vi "5ChPulserTrigsNew.vi"(1 "Motion Settings":T1={"No Motion?"=FALSE, "Motion System"=enum."NI 735x", "Motion Bd ID"=1, "Motion Profile"="SMAC1", "# Axis"=1, "Reverse Z axis?"=TRUE, "SMAC Axis"=0, "scan pair"=enum."y-(x) scan", "RT fps"=6.0, "Steps per mm"=[1000, 1000, 1000, 1000], "Motor Parameters"={"velocity ct/s"=[10000.0, 10000.0, 10000.0, 50000.0], "accel ct/s^2"=[50000.0, 50000.0, 50000.0, 200000.0]}, "One Way Scan"=FALSE, "Reverse One Way Scan"=FALSE, "Global Position (mm)"=[], "Plane"=0, "Distance between\nscan lines (um)"=0.0, "Distance between\nscan planes (um)"=0.0, "number of scan planes"=1, "Total steps in line"=0, "Xtra plane\ndistance  (um)"=100, "Xtra planes "=1, "Add Axis"=FALSE, "overshoot cts"=200, "BKPT Shift"=0, "Scan Start Time (ms)"=0, "ESP VISA"="GPIB::1::INSTR", "3rd Axis"=1, "GL Ref Out"=refnum, "Galil Address"=""} {"3rd Axis" items=["x", "y", "z", "w"]; "Xtra planes" min=1; "Xtra plane\ndistance  (um)" min=0; "Distance between\nscan planes (um)" format="%.2f"; "Distance between\nscan lines (um)" format="%.2f"; "SMAC Axis" items=["None"=0, "Axis 1"=1, "Axis 2"=2, "Axis 3"=3, "Axis 4"=4, "Axis 5"=5, "Axis 6"=6, "Axis 7"=7, "Axis 8"=8, "Vector Space 1"=17, "Vector Space 2"=18, "Vector Space 3"=19, "Vector Space 4"=20]; "Motion Bd ID" min=1 max=32 step=1}, 5 "Digitizer Settings":T5={"Digitizer delay (us) "=0.0, "rf points per line"=2048, "lines per plane"=128, "Samp Rate (Hz)"=100000000.0, "Additional dig delay (us)"=0.0, "Voltage Scale"=0.4, "Pre-Looks"=0, "Offset delay (us)"=0.0, "bits A/D"=8, "Avg Num"=1, "DigTimeOut"=5.0, "Rel Dig Delay"=0.0, "Dig Ch"=0, "LeCroyCluster"={"LeCroy Channels"=[TRUE, FALSE, FALSE, FALSE], "LC read pt offset"=0.0, "Sweep Avg"=FALSE}, "Main Digitizer"=enum."NI Digitizer", "Dig Config"=enum."Single channel", "Digitizer ID Cluster"={"Acqiris/Alazar/SP ID"=[], "NI Instr Handles"=[], "LeCroy VISA"="", "GaGe Handle"={"Handle"=0, "Sample size"=0, "Resolution"=0, "Offset"=0, "Channels"=0, "Boards"=0}, "ATS Ref"="ATS9350", "Acqiris Address"=["PCI::INSTR0"], "ADQRef"=refnum, "adq_cu_ptr"=refnum}, "Trigger Settings"={"Trig Source"=1, "Trig Coupling"=0, "Trig Slope"=0, "Level (mV)"=1500.0}, "Bulk Acq"=FALSE, "Bulk Start Indexes"=[], "Data Ref RF"=refnum, "NI ID/Channel"=[], "Total Dig CH"=1, "Xtra Ann Trig delay (us)"=10.0, "Fix Z Delay?"=FALSE, "One Way Transmission?"=FALSE, "Data Ref Log"=refnum} {"Trigger Settings"."Trig Slope" items=["Positive", "Negative"]; "Trigger Settings"."Level (mV)" format="%.2f"; "Trigger Settings"."Trig Coupling" items=["DC 1 MOhm", "AC 1 MOhm", "DC 50 Ohm", "AC 50 Ohm"]; "Trigger Settings"."Trig Source" items=["Chan 1", "External"]; "Rel Dig Delay" format="%.2f"; "DigTimeOut" format="%.2f"; "Avg Num" min=1; "Offset delay (us)" format="%.2f"; "Additional dig delay (us)" format="%.2f"; "Digitizer delay (us)" format="%.2f"}, 6 "XMIT":bool[](array[boolean])=[TRUE, TRUE, TRUE, TRUE, TRUE], 7 "high time":dbl=1e-06 format="%^.2e", 8 "Axis":u16(ring)=1 caption="Axis or Vector Space" items=["Axis 1"=1, "Axis 2"=2, "Axis 3"=3, "Axis 4"=4, "Axis 5"=5, "Axis 6"=6, "Axis 7"=7, "Axis 8"=8, "Vector Space 1"=17, "Vector Space 2"=18, "Vector Space 3"=19, "Vector Space 4"=20], 9 "M-mode?":bool, 10 "error in":errorcluster) -> (0 "5CH Pulser Tasks":refnum<k21>[](array[refnum]), 3 "error out":errorcluster)   [LabVIEW 2022 SP3]
uses:
  Digitizers/-DigitizerRoutines/DigitizerSettings.ctl
  Digitizers/-DigitizerRoutines/Digitizer.ctl
  Digitizers/-DigitizerRoutines/DigConfig.ctl
  Digitizers/-DigitizerRoutines/DigitizerID.ctl
  C:/Windows/System32/ADQAPI_dotNet_helper.dll
  Windows/System32/ADQAPI_dotNet_helper.dll
  Motion Controllers/NI_controller/-NI_MotionRoutines/MotionParameters.ctl
  Motion Controllers/NI_controller/-NI_MotionRoutines/MotionSys.ctl
  Motion Controllers/-MotionRoutines/ScanAxis.ctl
  Motion Controllers/-MotionRoutines/3rdAxis.ctl
  Switch Modules/SwitchGlobals.vi
  Motion Controllers/-MotionRoutines/MotionGlobals.vi
  <vilib>/DAQmx/create/channels.llb/DAQmx Create Channel (CO-Pulse Generation-Time).vi
  <vilib>/DAQmx/configure/trigger.llb/DAQmx Start Trigger (Digital Edge).vi
  PulserGlobals.vi
  <vilib>/DAQmx/create/channels.llb/DAQmx Create Channel (CO-Pulse Generation-Frequency).vi
  <vilib>/DAQmx/configure/timing.llb/DAQmx Timing (Implicit).vi
  <resource>/objmgr/daqmx.rc
panel:
  out "Array":dbl[](array[numeric]) format="%#_3e"
  in  "stop":bool
  # "Counter 1 output is the BNC on grey box."
  # "Trigger source comes from Gate of CTR0 (PFI9)\n\nThe NI trigger connector routes to CTR0 Gate"
  # "1-D and 2-D B scan settings"
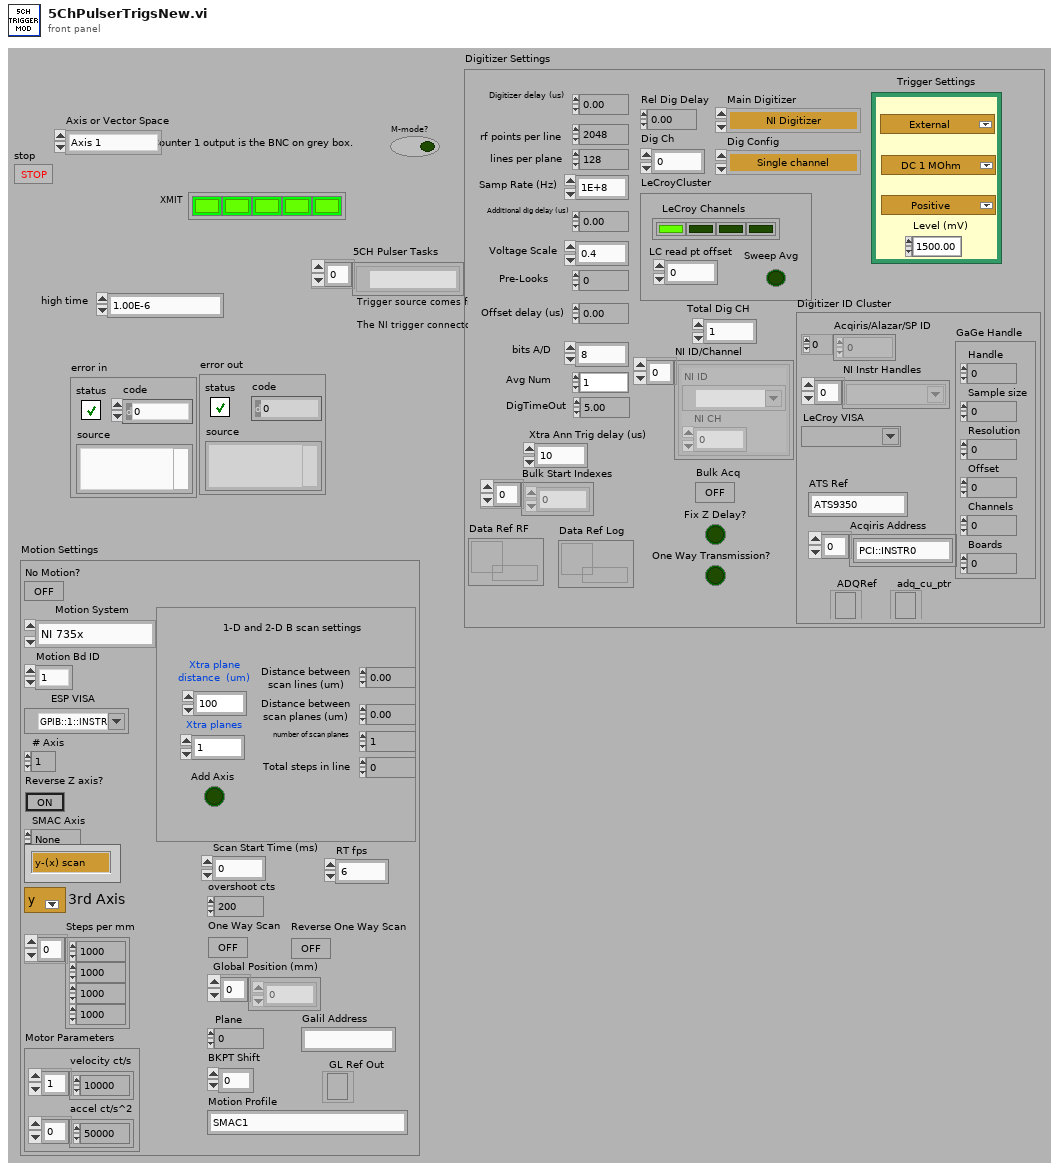
[diagram p1: front panel]
types:
  T1 = typedef "MotionParameters.ctl" = cluster{"No Motion?":bool, "Motion System":T2, "Motion Bd ID":u8, "Motion Profile":string, "# Axis":i8, "Reverse Z axis?":bool, "SMAC Axis":u16, "scan pair":T3, "RT fps":sgl, "Steps per mm":i32[], "Motor Parameters":cluster{"velocity ct/s":dbl[], "accel ct/s^2":dbl[]}, "One Way Scan":bool, "Reverse One Way Scan":bool, "Global Position (mm)":dbl[], "Plane":i32, "Distance between\nscan lines (um)":sgl, "Distance between\nscan planes (um)":sgl, "number of scan planes":i32, "Total steps in line":i32, "Xtra plane\ndistance  (um)":i32, "Xtra planes ":i32, "Add Axis":bool, "overshoot cts":i32, "BKPT Shift":i32, "Scan Start Time (ms)":u32, "ESP VISA":refnum<visa-resource-name>, "3rd Axis":T4, "GL Ref Out":refnum<k7>, "Galil Address":string}
  T2 = typedef "MotionSys.ctl" = enum16{"MM3000", "NI 735x", "Newport ESP", "No Motion Card", "Galil"}
  T3 = typedef "ScanAxis.ctl" = enum16{"y-(x) scan", "x-(y) scan", "z-(x) scan", "z-(y) scan", "y-(z) scan", "x-(z) scan", "w-(x) scan", "w-(y) scan", "w-(z) scan", "x-(w) scan", "y-(w) scan", "z-(w) scan"}
  T4 = typedef "3rdAxis.ctl" = u16
  T5 = typedef "DigitizerSettings.ctl" = cluster{"Digitizer delay (us) ":dbl, "rf points per line":i32, "lines per plane":i32, "Samp Rate (Hz)":dbl, "Additional dig delay (us)":dbl, "Voltage Scale":dbl, "Pre-Looks":i32, "Offset delay (us)":dbl, "bits A/D":i8, "Avg Num":i32, "DigTimeOut":sgl, "Rel Dig Delay":sgl, "Dig Ch":i32, "LeCroyCluster":cluster{"LeCroy Channels":bool[], "LC read pt offset":dbl, "Sweep Avg":bool}, "Main Digitizer":T6, "Dig Config":T7, "Digitizer ID Cluster":T8, "Trigger Settings":cluster{"Trig Source":u16, "Trig Coupling":u16, "Trig Slope":u16, "Level (mV)":dbl}, "Bulk Acq":bool, "Bulk Start Indexes":i32[], "Data Ref RF":refnum<data-value>, "NI ID/Channel":cluster{"NI ID":refnum<k15>, "NI CH":i32}[], "Total Dig CH":i32, "Xtra Ann Trig delay (us)":dbl, "Fix Z Delay?":bool, "One Way Transmission?":bool, "Data Ref Log":refnum<data-value>}
  T6 = typedef "Digitizer.ctl" = enum16{"Acqiris Digitizer", "NI Digitizer", "LeCroy", "GaGe", "AlazarTech", "No Digitizer", "Teledyne"}
  T7 = typedef "DigConfig.ctl" = enum16{"Single channel", "2 Chans w/ 2 Acqiris", "2 Chans w/ 1 Acqiris", "5-CH Pulser New", "5-CH pulser w/ ann array", "5-pass style ann array", "Empty"}
  T8 = typedef "DigitizerID.ctl" = cluster{"Acqiris/Alazar/SP ID":u32[], "NI Instr Handles":refnum<k15>[], "LeCroy VISA":refnum<visa-resource-name>, "GaGe Handle":cluster{"Handle":u32, "Sample size":u32, "Resolution":i32, "Offset":i32, "Channels":u32, "Boards":u32}, "ATS Ref":string, "Acqiris Address":string[], "ADQRef":refnum<k24>, "adq_cu_ptr":refnum<k24>}
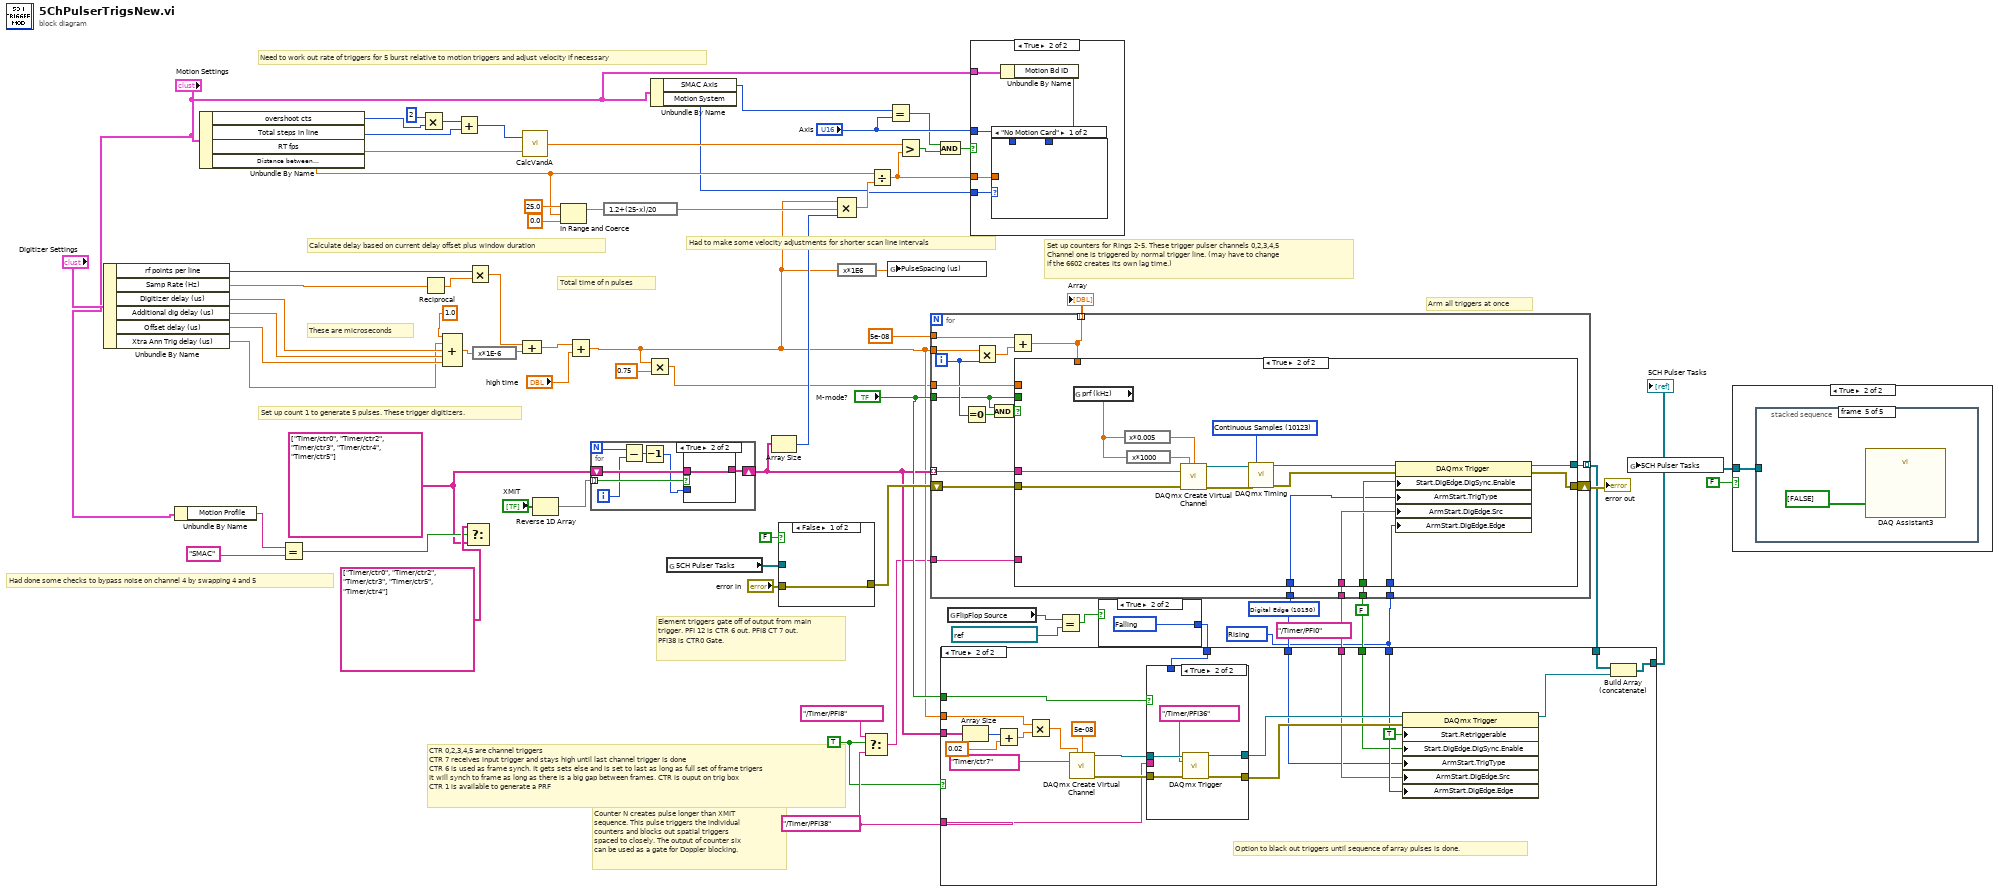
[diagram p0: block diagram]
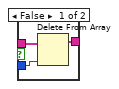
[diagram p2: hidden frame]
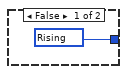
[diagram p3: hidden frame]
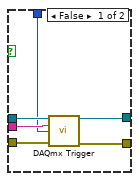
[diagram p5: hidden frame]
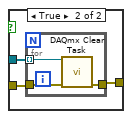
[diagram p6: hidden frame]
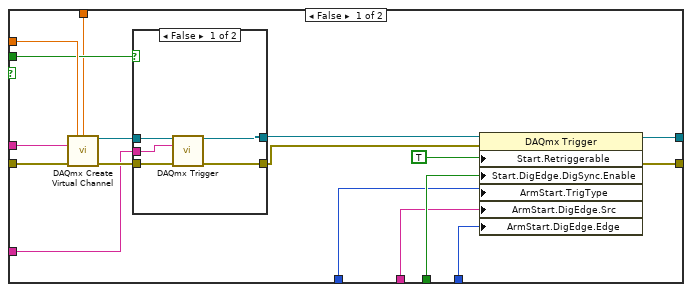
[diagram p7: hidden frame]
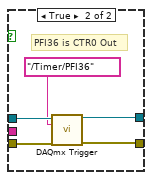
[diagram p8: hidden frame]
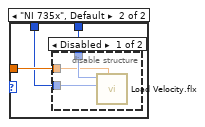
[diagram p10: hidden frame]
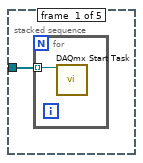
[diagram p13: hidden frame]
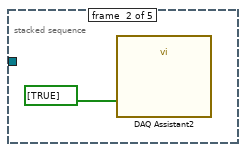
[diagram p14: hidden frame]
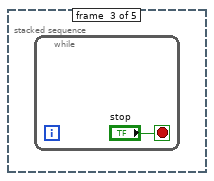
[diagram p15: hidden frame]
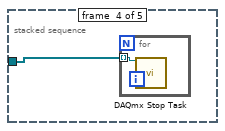
[diagram p16: hidden frame]
diagram:
  w22 = TRUE
  w23 = tag "/Timer/PFI38" ("Source")
  w35 = 10280 items=["Rising"=10280, "Falling"=10171] ("ArmStart.DigEdge.Edge")
  w41 = 10150 items=["Digital Edge"=10150, "None"=10230] ("ArmStart.TrigType")
  w43 = tag "/Timer/PFI0" ("ArmStart.DigEdge.Src")
  w1 = tag[] ["Timer/ctr0", "Timer/ctr2", "Timer/ctr3", "Timer/ctr4", "Timer/ctr5"]
  w42 = FALSE
  # "Had done some checks to bypass noise on channel 4 by swapping 4 and 5"
  # "CTR 0,2,3,4,5 are channel triggers\nCTR 7 receives input trigger and stays high until last channel trigger is done\nCTR 6 is used as frame synch. It gets sets else and is set to last as long as full set of frame trigers\nIt will synch to frame as long as there is a big gap between frames. CTR is ouput on trig box\nCTR 1 is available to generate a PRF"
  # "Counter N creates pulse longer than XMIT sequence. This pulse triggers the individual counters and blocks out spatial triggers spaced to closely. The output of counter six can be used as a gate for Doppler blocking."
  # "Element triggers gate off of output from main trigger. PFI 12 is CTR 6 out. PFI8 CT 7 out. PFI38 is CTR0 Gate."
  # "Arm all triggers at once"
  # "Had to make some velocity adjustments for shorter scan line intervals"
  # "Total time of n pulses"
  # "Need to work out rate of triggers for 5 burst relative to motion triggers and adjust velocity if necessary"
  # "Set up counters for Rings 2-5. These trigger pulser channels 0,2,3,4,5\nChannel one is triggered by normal trigger line. (may have to change \nif the 6602 creates its own lag time.)"
  # "Set up count 1 to generate 5 pulses. These trigger digitizers."
  # "Calculate delay based on current delay offset plus window duration"
  # "These are microseconds"
  n1 = Unbundle By Name("Digitizer Settings") -> ("rf points per line"=w20:i32, "Samp Rate (Hz)"=w19:dbl, "Digitizer delay (us)"=w18:dbl, "Additional dig delay (us)"=w17:dbl, "Offset delay (us)"=w16:dbl, "Xtra Ann Trig delay (us)"=w7:dbl)
  n2 = Unbundle By Name("Motion Settings") -> ("Motion Profile"=w3:string)
  n3 = Unbundle By Name("Motion Settings") -> ("overshoot cts"=w14:i32, "Total steps in line"=w13:i32, "RT fps"=w12:sgl, "Distance between\nscan lines (um)"=w11:sgl)
  n4 = Equal?(x=w3, y="SMAC" ("Motion Profile")) -> (x = y?=w2:bool)
  n5 = Multiply(x=2, y=w14) -> (x*y=w64:i32)
  n6 = Reciprocal(x=w19) -> (1/x=w70:dbl)
  n7 = Compound Arithmetic op=ADD(1.0 ("y"), w7, w18, w17, w16) -> (w52:dbl)
  n8 = Add(x=w64, y=w13) -> (x+y=w63:i32)
  n9 = Select(t=tag[] ["Timer/ctr0", "Timer/ctr2", "Timer/ctr3", "Timer/ctr5", "Timer/ctr4"], s=w2, f=w1) -> ()  [unwired: 1 out]
  n10 = Multiply(x=w20, y=w70) -> (x*y=w71:dbl)
  n11 = expression code="x*1E-6"(w52) -> (w51:dbl)
  n12 = call "CalcVandA.vi"("distance"=w63, "fps"=w12) -> ("Velocity"=w62:dbl)  [unwired: 2 out]
  n13 = Compound Arithmetic op=ADD(w71, w51) -> (w59:dbl)
  n14 = Reverse 1D Array(array="XMIT") -> (reversed array=w32:bool[])
  n15 = In Range and Coerce(upper limit=sgl 25.0, x=w11, lower limit=sgl 0.0) -> (coerced(x)=w58:sgl)  [unwired: 1 out]
  n16 = Add(x=w59, y="high time") -> (x+y=w29:dbl)
  n17 = for {
    N -> [w75]
    shift-right: [w76] -> w31
    shift-left: w1 -> [w77]
    tunnel: w32 -> [w78] mode=indexing
    i -> [w74]
    n18 = Subtract(x=w75, y=w74) -> (x-y=w73:i32)
    n19 = Decrement(x=w73) -> (x-1=w72:i32)
    n20 = case shown="True" w78 {
      tunnel: w77 -> [w81 w82]
      tunnel: [w80 w82] -> w76
      tunnel: w72 -> [w79 _]
      frame False {
        n21 = Delete From Array(array=w81, index=w79) -> (array with subset deleted=w80:tag[])  [unwired: 1 in, 1 out]
      }
      frame True {
      }
    }
  }
  n22 = expression code="1.2+(25-x)/20"(w58) -> (w55:sgl)
  n23 = Multiply(x=w29, y=0.75) -> (x*y=w27:dbl)
  n24 = Unbundle By Name("Motion Settings") -> ("SMAC Axis"=w10:u16, "Motion System"=w9:T2)
  n25 = global read "MotionGlobals.vi" "5CH Pulser Tasks"() -> (w67:refnum<k21>[])
  n26 = Array Size(array=w31) -> (size(s)=w30:i32)
  n27 = case shown="False" FALSE {
    tunnel: "error in" -> [w83 w86]
    tunnel: w67 -> [_ w85]
    tunnel: [w83 w84] -> w60
    frame False {
    }
    frame True {
      n28 = for {
        tunnel: [w89] -> w84
        tunnel: w85 -> [w88] mode=indexing
        tunnel: w86 -> [w87]
        n29 = call <vilib>:"DAQmx Clear Task.vi"("task in"=w88, "error in"=w87) -> ("error out"=w89:errorcluster)  [unwired: 13 out]
      }
    }
  }
  n30 = Compound Arithmetic op=MULTIPLY(w29, w55, w30) -> (w54:dbl)
  n31 = expression code="x*1E6"(w29) -> (w8:dbl)
  n32 = Select(t=tag "/Timer/PFI8" ("Source"), s=w22, f=w23) -> (s? t:f=w21:tag)
  n33 = Divide(x=w11, y=w54) -> (x/y=w61:dbl)
  n34 = Equal?(x=w10, y="Axis") -> (x = y?=w46:bool)
  n35 = global write "SwitchGlobals.vi" "PulseSpacing (us)"(w8) -> ()
  n36 = Greater?(x=w62, y=w61) -> (0:w48:bool)
  n37 = for {
    tunnel: w29 -> [w107]
    tunnel: w27 -> [w102]
    shift-right: [w104] -> w69
    shift-left: w60 -> [w106]
    tunnel: 5e-08 ("x") -> [w101]
    tunnel: w21 -> [w100]
    tunnel: w31 -> [w103] mode=indexing
    tunnel: [w99] -> w40 mode=indexing
    tunnel: "M-mode?" -> [w96]
    tunnel: w42 -> [w94]
    tunnel: w43 -> [w93]
    tunnel: w41 -> [w92]
    tunnel: w35 -> [w91]
    tunnel: [w90] -> w33 mode=indexing
    i -> [w97]
    n38 = Equal To 0?(x=w97) -> (x = 0?=w95:bool)
    n39 = Multiply(x=w107, y=w97) -> (x*y=w105:dbl)
    n40 = And(x=w96, y=w95) -> (x .and. y?=w98:bool)
    n41 = Add(x=w101, y=w105) -> (x+y=w90:dbl)
    n42 = case shown="True" w98 {
      tunnel: w106 -> [w124 w146]
      tunnel: [w122 w140] -> w104
      tunnel: w103 -> [w121 w147]
      tunnel: w102 -> [w119 _]
      tunnel: w100 -> [w118 _]
      tunnel: [w117 w142] -> w99
      tunnel: w96 -> [w116 _]
      tunnel: w90 -> [w115 _]
      tunnel: w94 -> [w113 w138]
      tunnel: w93 -> [w112 w139]
      tunnel: w92 -> [w109 w137]
      tunnel: w91 -> [w108 w136]
      frame False {
        n43 = call-poly <vilib>:"DAQmx Create Virtual Channel.vi"("high time"=w119, "low time"=w115, "counter"=w121, "error in"=w124) -> ("task out"=w120:refnum<k21>, "error out"=w123:errorcluster)  [unwired: 5 in, 5 out]
        n44 = case shown="False" w116 {
          tunnel: w123 -> [w128 w134]
          tunnel: w120 -> [w129 w133]
          tunnel: [w127 w132] -> w111
          tunnel: w118 -> [w125 _]
          tunnel: [w126 w130] -> w110
          frame False {
            n45 = call-poly <vilib>:"DAQmx Trigger.vi"("task/channels in"=w129, "source"=w125, "error in"=w128) -> ("task out"=w127:refnum<k21>, "error out"=w126:errorcluster)  [unwired: 2 in, 9 out]
          }
          frame True {
            # "PFI36 is CTR0 Out"
            n46 = call-poly <vilib>:"DAQmx Trigger.vi"("task/channels in"=w133, "source"=tag "/Timer/PFI36", "error in"=w134) -> ("task out"=w132:refnum<k21>, "error out"=w130:errorcluster)  [unwired: 1 in, 10 out]
          }
        }
        n47 = property class="DAQmx Trigger"(reference=w111, error in=w110, "Start.Retriggerable"=TRUE, "Start.DigEdge.DigSync.Enable"=w113, "ArmStart.TrigType"=w109, "ArmStart.DigEdge.Src"=w112, "ArmStart.DigEdge.Edge"=w108) -> (reference out=w117:refnum<k21>, error out=w122:errorcluster)
      }
      frame True {
        w150 = 10123 items=["Finite Samples"=10178, "Continuous Samples"=10123, "Hardware Timed Single Point"=12522] ("sample mode")
        n48 = global read "PulserGlobals.vi" "prf (kHz)"() -> (w135:dbl)
        n49 = expression code="x*0.005"(w135) -> (w145:dbl)
        n50 = expression code="x*1000"(w135) -> (w144:dbl)
        n51 = call-poly <vilib>:"DAQmx Create Virtual Channel.vi"("frequency"=w144, "duty cycle"=w145, "counter"=w147, "error in"=w146) -> ("task out"=w149:refnum<k21>, "error out"=w148:errorcluster)  [unwired: 5 in, 5 out]
        n52 = call-poly <vilib>:"DAQmx Timing.vi"("task/channels in"=w149, "sample mode"=w150, "error in"=w148) -> ("task out"=w143:refnum<k21>, "error out"=w141:errorcluster)  [unwired: 11 in]
        n53 = property class="DAQmx Trigger"(reference=w143, error in=w141, "Start.DigEdge.DigSync.Enable"=w138, "ArmStart.TrigType"=w137, "ArmStart.DigEdge.Src"=w139, "ArmStart.DigEdge.Edge"=w136) -> (reference out=w142:refnum<k21>, error out=w140:errorcluster)
      }
    }
  }
  "error out" <- w69
  "Array" <- w33
  n54 = And(x=w46, y=w48) -> (x .and. y?=w47:bool)
  n55 = global read "MotionGlobals.vi" "FlipFlop Source"() -> (w38:refnum<k21>)
  n56 = case shown="True" w47 {
    tunnel: w61 -> [_ w155]
    tunnel: "Axis" -> [_ w154]
    tunnel: w9 -> [_ w153]
    tunnel: "Motion Settings" -> [_ w152]
    frame False {
    }
    frame True {
      n57 = Unbundle By Name(w152) -> ("Motion Bd ID"=w151:u8)
      n58 = case shown="\"No Motion Card\"" w153 {
        tunnel: w151 -> [_ w158]
        tunnel: w155 -> [_ w157]
        tunnel: w154 -> [_ w156]
        frame "No Motion Card" {
        }
        frame "NI 735x", Default {
          n59 = disable-structure shown="Disabled" {
            disable-tunnel: w158 -> [w161 _]
            disable-tunnel: w157 -> [w160 _]
            disable-tunnel: w156 -> [w159 _]
            frame Disabled {
              n60 = call <vilib>:"Load Velocity.flx"("Velocity (10000)"=w160, "Axis or Vector Space"=w159, "Board ID"=w161) -> ()  [unwired: 1 in, 6 out]
            }
            frame Enabled {
            }
          }
        }
      }
    }
  }
  n61 = Equal?(x=w38, y=refnum<k21> "QuantFlipFlop" ("FlipFlop Source")) -> (x = y?=w36:bool)
  n62 = case shown="True" w36 {
    tunnel: [w162 w163] -> w26
    frame False {
      w162 = 10280 items=["Rising"=10280, "Falling"=10171] ("ArmStart.DigEdge.Edge")
    }
    frame True {
      w163 = 10171 items=["Rising"=10280, "Falling"=10171] ("ArmStart.DigEdge.Edge")
    }
  }
  n63 = case shown="True" w22 {
    tunnel: w23 -> [_ w185]
    tunnel: "M-mode?" -> [_ w184]
    tunnel: w35 -> [_ w181]
    tunnel: w43 -> [_ w180]
    tunnel: w42 -> [_ w179]
    tunnel: w41 -> [_ w177]
    tunnel: w29 -> [_ w170]
    tunnel: [w164 w173] -> w39
    tunnel: w40 -> [w164 w174]
    tunnel: w31 -> [_ w171]
    tunnel: w26 -> [_ w168]
    frame False {
    }
    frame True {
      # "Option to black out triggers until sequence of array pulses is done."
      n64 = Array Size(array=w171) -> (size(s)=w167:i32)
      n65 = Add(x=w167, y=0.02 ("x")) -> (x+y=w166:dbl)
      n66 = Multiply(x=w170, y=w166) -> (x*y=w169:dbl)
      n67 = call-poly <vilib>:"DAQmx Create Virtual Channel.vi"("high time"=w169, "low time"=5e-08 ("x"), "counter"=tag "Timer/ctr7" ("Counter(s)")) -> ("task out"=w187:refnum<k21>, "error out"=w186:errorcluster)  [unwired: 6 in, 5 out]
      n68 = case shown="True" w184 {
        tunnel: w187 -> [w193 w198]
        tunnel: [w192 w197] -> w183
        tunnel: [w191 w195] -> w182
        tunnel: w186 -> [w190 w194]
        tunnel: w185 -> [w189 _]
        tunnel: w168 -> [w188 _]
        frame False {
          n69 = call-poly <vilib>:"DAQmx Trigger.vi"("task/channels in"=w193, "source"=w189, "edge"=w188, "error in"=w190) -> ("task out"=w192:refnum<k21>, "error out"=w191:errorcluster)  [unwired: 1 in, 9 out]
        }
        frame True {
          n70 = call-poly <vilib>:"DAQmx Trigger.vi"("task/channels in"=w198, "source"=tag "/Timer/PFI36", "error in"=w194) -> ("task out"=w197:refnum<k21>, "error out"=w195:errorcluster)  [unwired: 1 in, 10 out]
        }
      }
      n71 = property class="DAQmx Trigger"(reference=w183, error in=w182, "Start.Retriggerable"=TRUE, "Start.DigEdge.DigSync.Enable"=w179, "ArmStart.TrigType"=w177, "ArmStart.DigEdge.Src"=w180, "ArmStart.DigEdge.Edge"=w181) -> (reference out=w172:refnum<k21>)  [unwired: 1 out]
      n72 = Build Array (concatenate)(w174, w172) -> (w173:refnum<k21>[])
    }
  }
  "5CH Pulser Tasks" <- w39
  n73 = global write "MotionGlobals.vi" "5CH Pulser Tasks"(w39) -> ()
  n74 = case shown="True" FALSE {
    tunnel: w39 -> [_ w199]
    frame False {
    }
    frame True {
      n75 = stacked-sequence {
        tunnel: w199 -> [w200 _ _ w204 _]
        frame #0 {
          n76 = for {
            tunnel: w200 -> [w201] mode=indexing
            n77 = call <vilib>:"DAQmx Start Task.vi"("task/channels in"=w201) -> ()  [unwired: 13 in, 2 out]
          }
        }
        frame #1 {
          n78 = call "DAQ Assistant2"("data"=bool[] [TRUE]) -> ()  [unwired: 17 in, 2 out]
        }
        frame #2 {
          n79 = while {
            stop <- "stop" stop-if-true
          }
        }
        frame #3 {
          n80 = for {
            tunnel: w204 -> [w205] mode=indexing
            n81 = call <vilib>:"DAQmx Stop Task.vi"("task/channels in"=w205) -> ()  [unwired: 13 in, 2 out]
          }
        }
        frame #4 {
          n82 = call "DAQ Assistant3"("data"=bool[] [FALSE]) -> ()  [unwired: 17 in, 2 out]
        }
      }
    }
  }
